vi "Polynomials.vi"() -> ()   [LabVIEW 2019]
panel:
  out "y":string
  in  "Opoznienie w [s]":dbl
  in  "STOP!!!!":bool
  in  "Enum":enum16{"Dziesietny", "Osemkowy", "Szesnastkowy"}(ring)
  in  "funkcja":bool
  in  "c":dbl
  in  "b":dbl
  in  "a":dbl
  in  "x":dbl
  # "y = a + bx + cx^2"
  # "y = a + bx^2 - 3x^4"
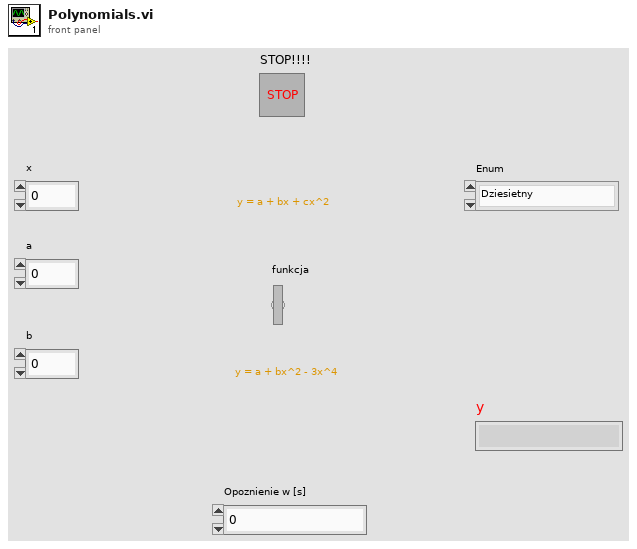
[diagram p1: front panel]
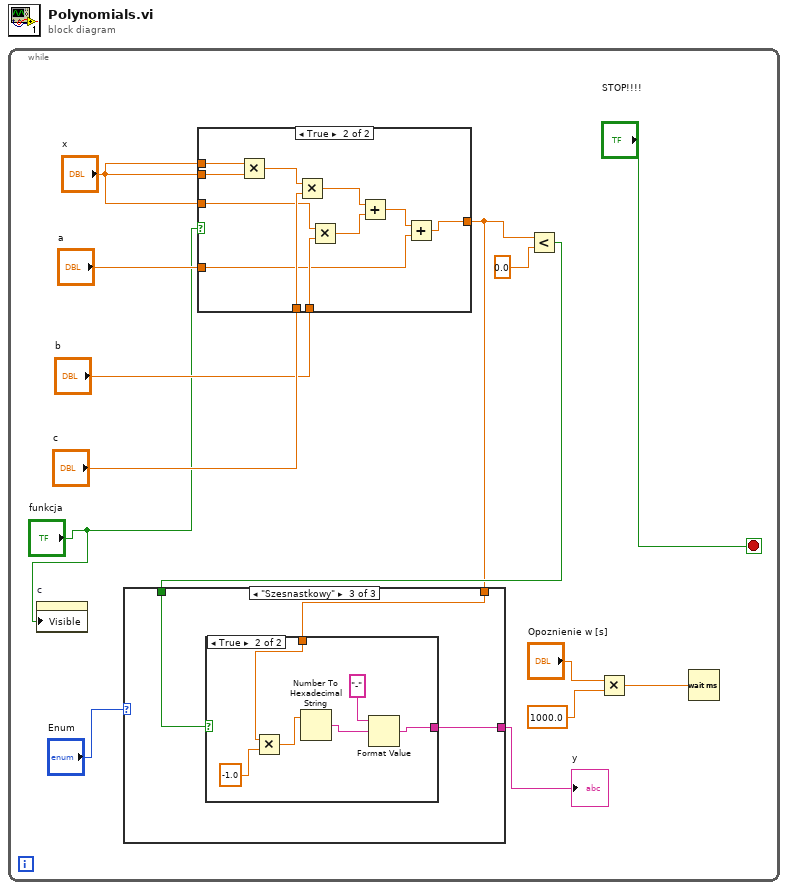
[diagram p0: block diagram]
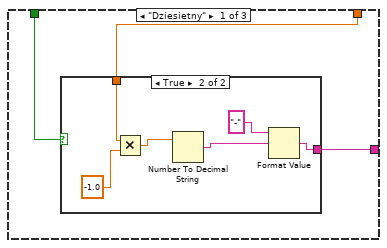
[diagram p2: hidden frame]
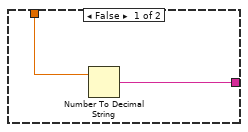
[diagram p3: hidden frame]
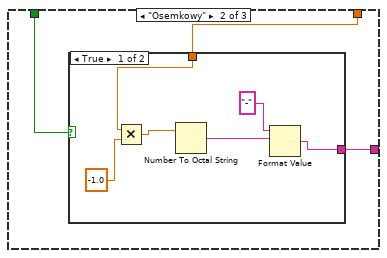
[diagram p4: hidden frame]
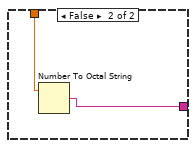
[diagram p5: hidden frame]
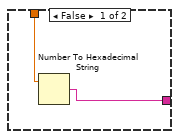
[diagram p6: hidden frame]
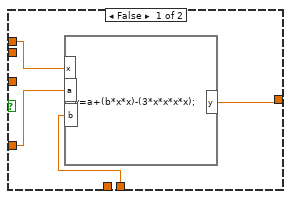
[diagram p7: hidden frame]
diagram:
  n1 = while {
    stop <- "STOP!!!!" stop-if-true
    n2 = property on="c" class="DigNum (strict)"("Visible"="funkcja") -> ()  [unwired: 2 in, 2 out]
    n3 = case shown="True" "funkcja" {
      tunnel: "x" -> [w51 w62]
      tunnel: "x" -> [_ w61]
      tunnel: "c" -> [_ w59]
      tunnel: "x" -> [_ w58]
      tunnel: "b" -> [w49 w57]
      tunnel: "a" -> [w50 w53]
      tunnel: [w48 w52] -> w3
      frame False {
        n4 = formula code="y=a+(b*x*x)-(3*x*x*x*x);"("x"=w51, "a"=w50, "b"=w49) -> ("y"=w48:dbl)
      }
      frame True {
        n5 = Multiply(x=w62, y=w61) -> (x*y=w60:dbl)
        n6 = Multiply(x=w60, y=w59) -> (x*y=w56:dbl)
        n7 = Multiply(x=w58, y=w57) -> (x*y=w55:dbl)
        n8 = Add(x=w56, y=w55) -> (x+y=w54:dbl)
        n9 = Add(x=w54, y=w53) -> (x+y=w52:dbl)
      }
    }
    n10 = Less?(x=w3, y=0.0) -> (x < y?=w4:bool)
    n11 = case shown="\"Szesnastkowy\"" "Enum" {
      tunnel: w4 -> [w17 w28 w39]
      tunnel: w3 -> [w15 w27 w37]
      tunnel: [w16 w26 w38] -> w2
      frame "Dziesietny" {
        n12 = case shown="True" w17 {
          tunnel: [w19 w20] -> w16
          tunnel: w15 -> [w18 w24]
          frame False {
            n13 = Number To Decimal String(number=w18) -> (decimal integer string=w19:string)  [unwired: 1 in]
          }
          frame True {
            n14 = Multiply(x=w24, y=-1.0) -> (x*y=w23:dbl)
            n15 = Number To Decimal String(number=w23) -> (decimal integer string=w21:string)  [unwired: 1 in]
            n16 = Format Value(string ("")="-", format string=w21) -> (output string=w20:string)  [unwired: 1 in]
          }
        }
      }
      frame "Osemkowy" {
        n17 = case shown="True" w28 {
          tunnel: w27 -> [w33 w36]
          tunnel: [w31 w35] -> w26
          frame True {
            n18 = Multiply(x=w33, y=-1.0) -> (x*y=w32:dbl)
            n19 = Number To Octal String(2:w32) -> (0:w29:string)  [unwired: 1 in]
            n20 = Format Value(string ("")="-", format string=w29) -> (output string=w31:string)  [unwired: 1 in]
          }
          frame False {
            n21 = Number To Octal String(2:w36) -> (0:w35:string)  [unwired: 1 in]
          }
        }
      }
      frame "Szesnastkowy" {
        n22 = case shown="True" w39 {
          tunnel: [w41 w44] -> w38
          tunnel: w37 -> [w40 w46]
          frame False {
            n23 = Number To Hexadecimal String(2:w40) -> (0:w41:string)  [unwired: 1 in]
          }
          frame True {
            n24 = Multiply(x=w46, y=-1.0) -> (x*y=w45:dbl)
            n25 = Number To Hexadecimal String(2:w45) -> (0:w42:string)  [unwired: 1 in]
            n26 = Format Value(string ("")="-", format string=w42) -> (output string=w44:string)  [unwired: 1 in]
          }
        }
      }
    }
    "y" <- w2
    n27 = Multiply(x="Opoznienie w [s]", y=1000.0) -> (x*y=w7:dbl)
    n28 = Wait (ms)(milliseconds to wait=w7) -> ()  [unwired: 1 out]
  }
